vi "清晰度.vi"(0 "Image Pixels":u16[][](array[numeric]), 1 "path in":path, 4 "heigth":i32, 5 "width":i32, 7 "T":i32, 9 "error in (no error)":errorcluster, 13 "method":i32) -> (11 "error out":errorcluster, 14 "return type":dbl)   [LabVIEW 2016]
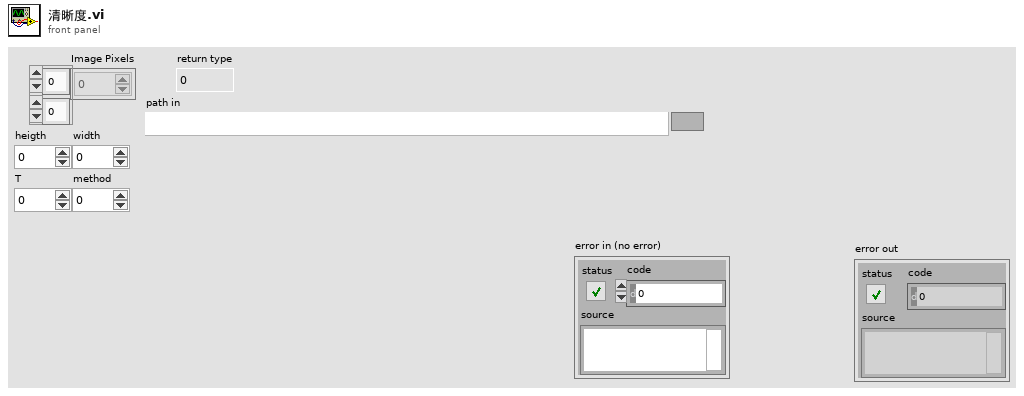
[diagram p1: front panel]
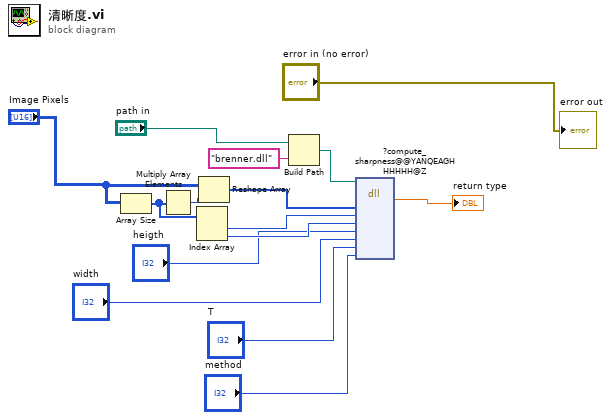
[diagram p0: block diagram]
diagram:
  n1 = Array Size(array="Image Pixels") -> (size(s)=w13:i32[])
  n2 = Multiply Array Elements(1:w13) -> (0:w10:i32)
  n3 = Index Array(array=w13) -> (element #1=w12:i32, element #2=w14:i32)  [unwired: 2 in]
  n4 = Reshape Array("Image Pixels", w10) -> (w11:u16[])
  n5 = Build Path(base path="path in", name or relative path="brenner.dll") -> (appended path=w6:path)
  n6 = dll-call lib="PTH2;abs DP2、Tiny1C程序测试标定databrenner.dll" fn="?compute_sharpness@@YANQEAGHHHHHH@Z"(path in=w6, "14"=w11, "rows"=w12, "cols"=w14, "heigth"="heigth", "width"="width", "T"="T", "method"="method") -> ("return type"=→"return type":dbl)  [unwired: 9 in, 2 out]
  "error out" <- "error in (no error)"
